vi "Delete DUT Connector.vi"(8 "error in (no error)":errorcluster, 9 "Connector (\"Connector1\")":string="Connector1", 10 "DUT (\"DUT1\")":string="DUT1", 11 "VISA resource name":refnum<visa-resource-name>) -> (0 "error out":errorcluster, 3 "VISA resource name out":refnum<visa-resource-name>)   [LabVIEW 2015, in "Rohde&Schwarz CMXP Base.lvlib"]
doc: "Deletes an antenna connector of the inactive DUT.\n\nAttribute:\n-\n\nRemote-control command:\nDELete:DUT:PROFile:CONNector"
uses:
  <instrlib>/Rohde&Schwarz CMXP Base/Rohde&Schwarz CMXP Base.lvlib
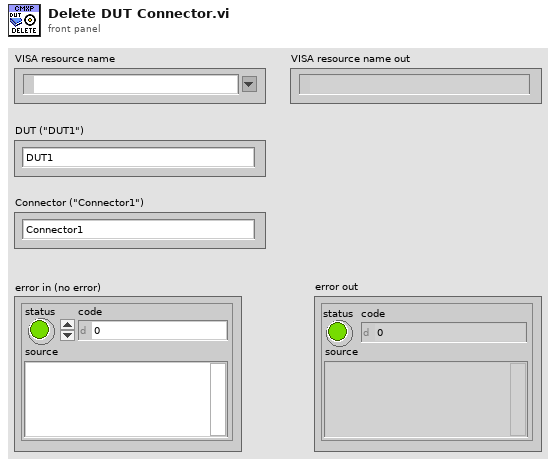
[diagram p1: front panel]
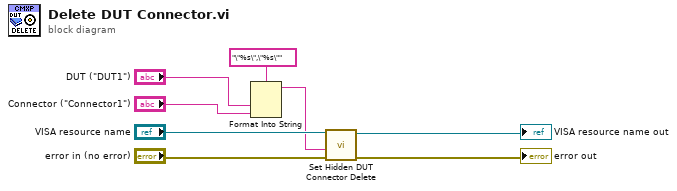
[diagram p0: block diagram]
diagram:
  n1 = Format Into String(format string="\"%s\",\"%s\"", "DUT (\"DUT1\")", "Connector (\"Connector1\")") -> (resulting string=w1:string)  [unwired: 2 in, 1 out]
  n2 = call "Set Hidden DUT Connector Delete"("error in (no error)"="error in (no error)", "Hidden DUT Connector Delete ()"=w1, "instrument handle"="VISA resource name") -> ("error out"=→"error out":errorcluster, "instrument handle out"=→"VISA resource name out":refnum<visa-resource-name>)  [unwired: 7 in]
